vi "System_Identify.vi"(3 "Samples Before Frequency Change":i32[](array[numeric]), 4 "Samples for Calculation":i32[](array[numeric]), 5 "Samples Before Measuring":i32[](array[numeric]), 6 "Frequency Responses":T1, 7 "In Frequency Sinusoids":cluster{"cos(wt)":dbl, " sin(wt)":dbl}, 8 "Current Sample":i32, 9 "Current Frequency Index":i32) -> (0 "Push To Plot":bool, 1 "System Phase":dbl, 2 "System Magnitude":dbl)   [LabVIEW 2013]
doc: "Over a given number of cycles, calculates the magnitude and phase of the frequency response of the system.\n\nTo calculate the magnitude and phase of the frequncy response at a given frequency, the following steps are taken:\n\n 1.) The phase and magnitude for the system response at different points in the system are measured.\n These are measured by a sub vi called Channel_Indentity.vi within this vi.\n\n CH0 = TF Intput | CH1 = TF Output\n\n 2.) From the magnitudes of these two response, the magnitude of the system's response is found:\n\n Sys_Mag = CH1_Mag / CH0_Mag\n\n 3.) From the phases of these two responses, the phase of the system's response is found:\n\n Sys+Phase = CH1_Phase - CH0_ Phase\n\nInputs: \n\n- Samples Before Measuring: A list of the last sample to be ignored for a given frequency. Following this sample, measuring should begin for a particular frequency.\n\n- Current Frequency Index: The index of the frequency which the freuency response (sinusoid) entered has.\n\n- Current Sample: The current sample being measured of the excited system. \n NOTE: Since we must excite the system before recording data, this will be the number of iterations the loop containing this function has run minus one.\n\n- In Frequency Sinusoids: A sine and cosine wave at the current excitation's frequency used to demodulate the system's frequency response to pull out the phase and magnitude.\n\n- Frequency Response: A cluster of the sinusoid responses of the system at two points to the DSA's output excitation at the previous time step. The Channel 0 response should be the system's input and the Channel 1 response should be the system's output.\n\n- Samples for Calculation: A list of the number of samples to be measured per frequency to measure the frequency response.\n\nOutputs: \n\n- System Magnitude: The magnitude of the system's frequncy response for a given frequency.\nNOTE: This value is only accurate once this vi has averaged all the number of input samples of the Channel 0 and Channel 1 frequency responses over a given amount of full cycles.\n\n- System Phase: The phase of the system's frequncy response for a given frequency.\nNOTE: This value is only accurate once this vi has averaged all the number of input samples of the Channel 0 and Channel 1 frequency responses over a given amount of full cycles.\n\n- Push to Plot: TRUE if the current sample is the last sample before a frequency cahnge, indicating it is the last sampled needed to be averaged and thus the following magnitude and phase output are accurate and should be pushed to the bode plot."
panel:
  out "System Initalize":bool
  out "CH1 Initalize":bool
  out "CH0 Initalize":bool
  out "CH1 Phase":dbl
  out "CH0 Phase":dbl
  out "CH1 Magnitude":dbl
  out "CH0 Magnitude":dbl
  # "System_Identify"
  # "System Inputs"
  # "Measurement Properties"
  # "Iteration Control"
  # "Frequency Response Components"
  # "Initalize Check"
  # "Magnitude"
  # "Phase"
  # "Send Data to Bode Plot?"
  # "Frequency Change"
  # "Per Frequency"
  # "Measuring"
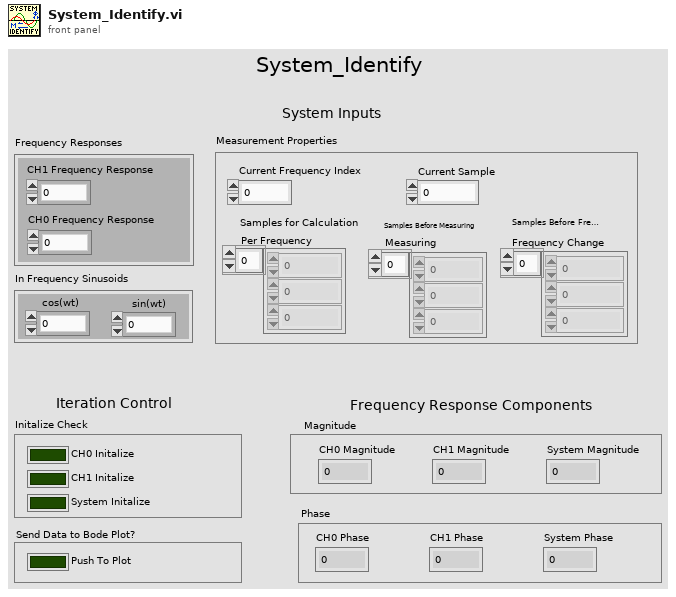
[diagram p1: front panel]
types:
  T1 = cluster{"CH1 Frequency Response":dbl, "CH0 Frequency Response":dbl}
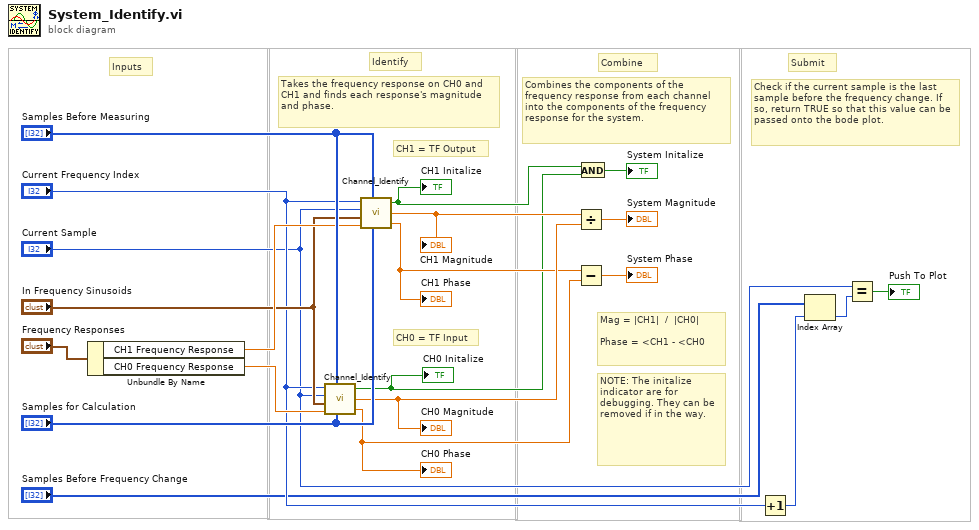
[diagram p0: block diagram]
diagram:
  # "Mag = |CH1|  /  |CH0|\n\nPhase = <CH1 - <CH0"
  # "CH1 = TF Output"
  # "CH0 = TF Input"
  # "NOTE: The initalize indicator are for debugging. They can be removed if in the way."
  # "Check if the current sample is the last sample before the frequency change. If so, return TRUE so that this value can be passed onto the bode plot."
  # "Submit"
  # "Combines the components of the frequency response from each channel into the components of the frequency response for the system."
  # "Combine"
  # "Takes the frequency response on CH0 and CH1 and finds each response's magnitude and phase."
  # "Identify"
  # "Inputs"
  n1 = Unbundle By Name("Frequency Responses") -> ("CH1 Frequency Response"=w19:dbl, "CH0 Frequency Response"=w18:dbl)
  n2 = call "Channel_Identify.vi"("Current Frequency Index"="Current Frequency Index", "Samples Before Measuring"="Samples Before Measuring", "Current Sample"="Current Sample", "In Frequency Sinusoids"="In Frequency Sinusoids", "Samples for Calculation"="Samples for Calculation", "Frequency Response"=w18) -> ("Initalize"=w11:bool, "Frequency Response Magnitude"=w14:dbl, "Frequency Response  Phase"=w12:dbl)
  "CH0 Magnitude" <- w14
  "CH0 Phase" <- w12
  "CH0 Initalize" <- w11
  n3 = call "Channel_Identify.vi"("Current Frequency Index"="Current Frequency Index", "Samples Before Measuring"="Samples Before Measuring", "Current Sample"="Current Sample", "In Frequency Sinusoids"="In Frequency Sinusoids", "Samples for Calculation"="Samples for Calculation", "Frequency Response"=w19) -> ("Initalize"=w3:bool, "Frequency Response Magnitude"=w15:dbl, "Frequency Response  Phase"=w13:dbl)
  "CH1 Magnitude" <- w15
  "CH1 Phase" <- w13
  "CH1 Initalize" <- w3
  n4 = Divide(x=w15, y=w14) -> (x/y=→"System Magnitude":dbl)
  n5 = Subtract(x=w13, y=w12) -> (x-y=→"System Phase":dbl)
  n6 = And(x=w3, y=w11) -> (x .and. y?=→"System Initalize":bool)
  n7 = Increment(x="Current Frequency Index") -> (x+1=w7:i32)
  n8 = Index Array(array="Samples Before Frequency Change", index=w7) -> (element=w5:i32)
  n9 = Equal?(x="Current Sample", y=w5) -> (x = y?=→"Push To Plot":bool)
